vi "gyro -- async fitter.vi"(11 "server event pair":T9) -> ()   [LabVIEW 2020]
uses:
  lorentzian.ctl
  circle corners.ctl
  peak -- parameters -- complex fit.ctl
  wavepacket.ctl
  filter method control.ctl
  show-win- control.ctl
  server talk-to-back pair.ctl
  server talkback message type.ctl
  server talkto message type.ctl
  cwin.ctl
  plot refs -- filter related.ctl
  cursor window action.ctl
  publisher action.ctl
  cursor action.ctl
  2Dwindow.ctl
  filter - complex - four.vi
  linear interp iiii- complex - z-omega.vi
  peak -- PM find lorenzian - V3.vi
  tale of three indices.vi
  Q -- check range -- i -- real.vi
  filter -- window span logic.vi
  linear interp iiii- complex - z-omega - divide.vi
  linear interpolation iiii- complex.vi
  containing bix.vi
  <vilib>/Analysis/baseanly.llb/A x B.vi
  <vilib>/Analysis/baseanly.llb/Complex A x B.vi
  line -- complex.vi
  Q -- check range -- i -- integer.vi
  peak -- guess at omega -- dzdomega V2.vi
  command stack.vi
  tale of three indices -- check state.vi
  Q - not nan -- real.vi
  Q - not nan -- integer.vi
  peak -- z center from mult phase points.vi
  peak -- estimate for lorentzian.vi
  peak -- fake phase around center.vi
  peak -- get weights.vi
  peak -- four corner circle transformation logic.vi
  peak - fit phase around center - V2.vi
  array - generate range.vi
  circle center from three points.vi
  <vilib>/Utility/error.llb/Clear Errors.vi
  peak -- fit function -- minus arctan.vi
  <vilib>/Analysis/Matrix/Numeric/Conversions/Array To Matrix.vi
  <vilib>/Analysis/Matrix/Numeric/Conversions/Array To Matrix - RA2.vi
  <vilib>/Analysis/baseanly.llb/Inverse Matrix.vi
  <vilib>/Analysis/baseanly.llb/Real Inverse Matrix.vi
  <vilib>/gmath/NumericalOptimization/Nonlinear Curve Fit.vi
  <vilib>/gmath/NumericalOptimization/Nonlinear Curve Fit LM.vi
  KM_filter pipe - plot staff - more - V3.vi
panel:
  in  "Tab :  Fit controls":T1(tab)
  out "lorentzian":T2={"A (VHz)"=nan, "f (Hz)"=0.0, "G (Hz)"=0.0, "phi(rad)"=nan, "Q"=nan, "Norm  Ampl"=nan, "bg (V)"=nan+nani, "4corners"={"z (-pi/2)"=nan+nani, "z(inf)"=nan+nani, "z (pi/2)"=nan+nani, "z center"=nan+nani, "z(0)"=nan+nani, "radius"=nan}} {"bg (V)" format="%#9_9f"; "Q" format="%#9_9f"; "phi(rad)" format="%#9_9f"; "G (Hz)" format="%#9_9f"; "f (Hz)" format="%#9_9f"}
  in  "Plot: fragment - filter":cluster{dbl[], dbl[]}[](graph)=[{[], []}, {[], []}, {[], []}, {[], []}]
  out "Plot: phase around center":cluster{dbl[], dbl[]}[](graph)
  out "Plot: fragment":cluster{dbl[], dbl[]}[](graph)
  out "Plot: complex plane":cluster{dbl[], dbl[]}[](graph)=[{[], []}, {[nan, nan, nan, nan, nan, nan, nan, nan, nan, nan, nan, nan, nan, nan, nan, nan, nan, nan, nan, nan, nan, nan, nan, nan, nan, nan, nan, nan, nan, nan, nan, nan, nan, nan, nan, nan, nan, nan, nan, nan, nan, nan, nan, nan, nan, nan, nan, nan, nan, nan], [nan, nan, nan, nan, nan, nan, nan, nan, nan, nan, nan, nan, nan, nan, nan, nan, nan, nan, nan, nan, nan, nan, nan, nan, nan, nan, nan, nan, nan, nan, nan, nan, nan, nan, nan, nan, nan, nan, nan, nan, nan, nan, nan, nan, nan, nan, nan, nan, nan, nan]}, {[nan, nan, nan, nan, nan, nan, nan, nan, nan, nan, nan, nan, nan, nan, nan, nan, nan, nan, nan, nan], [nan, nan, nan, nan, nan, nan, nan, nan, nan, nan, nan, nan, nan, nan, nan, nan, nan, nan, nan, nan]}, {[nan, nan, nan, nan, nan, nan, nan, nan, nan, nan, nan, nan, nan, nan, nan, nan, nan, nan, nan, nan], [nan, nan, nan, nan, nan, nan, nan, nan, nan, nan, nan, nan, nan, nan, nan, nan, nan, nan, nan, nan]}, {[nan, nan, nan, nan, nan, nan, nan, nan, nan, nan, nan, nan, nan, nan, nan, nan, nan, nan, nan, nan], [nan, nan, nan, nan, nan, nan, nan, nan, nan, nan, nan, nan, nan, nan, nan, nan, nan, nan, nan, nan]}, {[nan, nan, nan, nan, nan, nan, nan, nan, nan, nan, nan, nan, nan, nan, nan, nan, nan, nan, nan, nan], [nan, nan, nan, nan, nan, nan, nan, nan, nan, nan, nan, nan, nan, nan, nan, nan, nan, nan, nan, nan]}, {[], []}]
  in  "scale gauge: Plot: complex plane":dbl(slide)=0.00275 min=0.0 max=0.3 step=1e-06 scale=1e-05..0.5 scale format="%#_3p"
  out "Plot: phase":cluster{"omega out":dbl[], dbl[]}(graph)
  out "Plot: win omega":T4(graph)
  out "Plot: dz/domega":cluster{"omega out":dbl[], dbl[]}(graph)
  in  "Plot: complex plane - filter":cluster{dbl[], dbl[]}[](graph)=[{[], []}, {[], []}, {[0.0, 0.0, 0.0, 0.0, 0.0, 0.0, 0.0, 0.0, 0.0, 0.0, 0.0, 0.0, 0.0, 0.0, 0.0, 0.0, 0.0, 0.0, 0.0, 0.0, 0.0, 0.0, 0.0, 0.0, 0.0, 0.0, 0.0, 0.0, 0.0, 0.0, 0.0, 0.0, 0.0, 0.0, 0.0, 0.0, 0.0, 0.0, 0.0, 0.0, 0.0, 0.0, 0.0, 0.0, 0.0, 0.0, 0.0, 0.0, 0.0, 0.0, 0.0, 0.0, 0.0, 0.0, 0.0, 0.0, 0.0, 0.0, 0.0, 0.0, 0.0, 0.0, 0.0, 0.0, 0.0, 0.0, 0.0, 0.0, 0.0, 0.0, 0.0, 0.0, 0.0, 0.0, 0.0, 0.0, 0.0, 0.0, 0.0, 0.0, 0.0, 0.0, 0.0, 0.0, 0.0, 0.0, 0.0, 0.0, 0.0, 0.0, 0.0, 0.0, 0.0, 0.0, 0.0, 0.0, 0.0, 0.0, 0.0, 0.0], [0.0, 0.0, 0.0, 0.0, 0.0, 0.0, 0.0, 0.0, 0.0, 0.0, 0.0, 0.0, 0.0, 0.0, 0.0, 0.0, 0.0, 0.0, 0.0, 0.0, 0.0, 0.0, 0.0, 0.0, 0.0, 0.0, 0.0, 0.0, 0.0, 0.0, 0.0, 0.0, 0.0, 0.0, 0.0, 0.0, 0.0, 0.0, 0.0, 0.0, 0.0, 0.0, 0.0, 0.0, 0.0, 0.0, 0.0, 0.0, 0.0, 0.0, 0.0, 0.0, 0.0, 0.0, 0.0, 0.0, 0.0, 0.0, 0.0, 0.0, 0.0, 0.0, 0.0, 0.0, 0.0, 0.0, 0.0, 0.0, 0.0, 0.0, 0.0, 0.0, 0.0, 0.0, 0.0, 0.0, 0.0, 0.0, 0.0, 0.0, 0.0, 0.0, 0.0, 0.0, 0.0, 0.0, 0.0, 0.0, 0.0, 0.0, 0.0, 0.0, 0.0, 0.0, 0.0, 0.0, 0.0, 0.0, 0.0, 0.0]}, {[0.0, 0.0, 0.0], [0.0, 0.0, 0.0]}, {[nan, nan, nan, nan, nan, nan, nan, nan, nan, nan, nan, nan, nan, nan, nan, nan, nan, nan, nan, nan], [nan, nan, nan, nan, nan, nan, nan, nan, nan, nan, nan, nan, nan, nan, nan, nan, nan, nan, nan, nan]}, {[0.0, 0.0, 0.0, 0.0, 0.0, 0.0, 0.0, 0.0, 0.0, 0.0, 0.0, 0.0, 0.0, 0.0, 0.0, 0.0, 0.0, 0.0, 0.0, 0.0], [0.0, 0.0, 0.0, 0.0, 0.0, 0.0, 0.0, 0.0, 0.0, 0.0, 0.0, 0.0, 0.0, 0.0, 0.0, 0.0, 0.0, 0.0, 0.0, 0.0]}]
  in  "parameters -- scan monitor control.ctlparameters: complex fit":T5={"main VI path"=path "", "scale factor"=3.0, "# of grid points"=200, "parameters: wavepacket"={"R"=0.5, "wave number"=22.0, "delta k"=7.0, "radii vector"=[], "radial section"=[], "wave vector"=22.0, "wavepacket is"=TRUE}, "span"=0.27789, "interference ?"=enum."cp z center", "filter method"=enum."three"} {"span" min=0.0 max=0.5 step=1e-05 scale=0.0001..0.5 scale format="%#_5f"; "parameters: wavepacket"."delta k" format="%#_3f"; "parameters: wavepacket"."wave number" format="%#_3f"; "parameters: wavepacket"."R" format="%#_3f"}
  in  "win":T8={"cen (Hz)"=45005.0594236074, "win (Hz)"=127.23590686512762, "left (Hz)"=44941.44147017484, "right (Hz)"=45068.67737703997}
  out "circle frequency (Hz)":dbl format="%#11_11f"
  out "circle gamma (Hz)":dbl format="%#11_11f"
  out "circle phase (rad)":dbl=nan format="%#11_11f"
  out "circle Q":dbl=nan format="%#11_11f"
  in  "use fast fit!":bool
  in  "plot staff!":enum16{"plot", "do not plot", "a"}(ring)
  in  "tab":enum32{"complex plane"}(tab)
  in  "Ignore win":T10={"cen (Hz)"=0.0, "win (Hz)"=0.0, "left (Hz)"=-8.969831627629043, "right (Hz)"=8.26461485679713}
  out "# of points":dbl=953.475933538175
  out "center (kHz)":dbl=3399.029286744401
  out "win width (kHz)":dbl=76.27809365793496
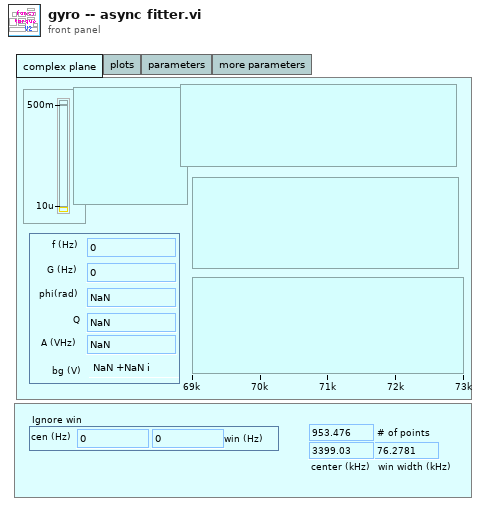
[diagram p1: front panel]
types:
  T1 = enum32{"complex plane", "plots", "parameters", "more parameters"}
  T2 = typedef "lorentzian.ctl" = cluster{"A (VHz)":dbl, "f (Hz)":dbl, "G (Hz)":dbl, "phi(rad)":dbl, "Q":dbl, "Norm  Ampl":dbl, "bg (V)":cdb, "4corners":T3}
  T3 = typedef "circle corners.ctl" = cluster{"z (-pi/2)":cdb, "z(inf)":cdb, "z (pi/2)":cdb, "z center":cdb, "z(0)":cdb, "radius":dbl}
  T4 = cluster{"omega out":dbl[], "win omega out":dbl[]}
  T5 = typedef "peak -- parameters -- complex fit.ctl" = cluster{"main VI path":path, "scale factor":dbl, "# of grid points":i32, "parameters: wavepacket":T6, "span":dbl, "interference ?":enum16{"cp z center", "pm zcenter", "fancy"}, "filter method":T7}
  T6 = typedef "wavepacket.ctl" = cluster{"R":dbl, "wave number":dbl, "delta k":dbl, "radii vector":dbl[], "radial section":cdb[], "wave vector":dbl, "wavepacket is":bool}
  T7 = typedef "filter method control.ctl" = enum16{"four", "five", "one", "two", "three", "zero", "minus one", "minus two"}
  T8 = typedef "show-win- control.ctl" = cluster{"cen (Hz)":dbl, "win (Hz)":dbl, "left (Hz)":dbl, "right (Hz)":dbl}
  T9 = typedef "server talk-to-back pair.ctl" = cluster{"talkback event":refnum<user-event>, "talkto event":refnum<user-event>}
  T10 = typedef "cwin.ctl" = cluster{"cen (Hz)":dbl, "win (Hz)":dbl, "left (Hz)":dbl, "right (Hz)":dbl}
  T11 = typedef "plot refs -- filter related.ctl" = cluster{"Plot: complex plane - filter":refnum<vi>, "Plot: dz/domega":refnum<vi>, "Plot: fragment filter":refnum<vi>, "Plot: win omega":refnum<vi>, "Plot: phase":refnum<vi>, "Plot: phase around center":refnum<vi>, "Plot: complex plane":refnum<vi>, "Plot: fragment":refnum<vi>}
  T12 = typedef "cursor window action.ctl" = enum16{"balance", "h. offset change", "cursor moves", "change center", "change window", "init", "check", "reset", "set y to middle", "idle", "-write all Y", "-write left.X", "-write center.X", "-write right.X", "-write all X", "-change center", "-change window", "-change skew", "-read cursor 2", "-read cursor 1", "-read cursor 0", "-read all cursors", "-reset", "-read plot scale", "-set y to middle", "-Q: center.Y is visible", "-Q: window is visible", "-parse center.Y", "-right left from center", "-left move", "-right move", "-set center.Y", "-empty", "-set cursors to default", "-check", "-write center.Y", "-copy cursor 1", "-copy cursor 0", "-copy cursor 2", "move right", "move left", "shrink", "broaden", "skew up", "skew down", "-write plot scale", "zoom X", "change cen&win", "zoom to all data", "color--red", "color--green", "color--yellow", "read", "zoom out", "zoom in", "slide right", "slide left", "set range aspect ratio to 1"}
  T13 = typedef "eventvkey.ctl" = enum16{"ASCII", "Enter", "Return", "Shift", "Ctrl", "Alt", "Cmd", "Opt", "Caps", "NumLock", "Clear", "Break", "Up", "Down", "Left", "Right", "Insert", "Delete", "Home", "End", "PageUp", "PageDown", "Escape", "Help", "Pause", "ScrollLock", "F1", "F2", "F3", "F4", "F5", "F6", "F7", "F8", "F9", "F10", "F11", "F12", "F13", "F14", "F15", "F16", "F17", "F18", "F19", "F20", "F21", "F22", "F23", "F24", "Play", "VolumeUp", "VolumeDown", "Mute", "Two Byte Char"}
  T14 = typedef "publisher action.ctl" = enum16{"set", "get", "init", "check"}
  T15 = typedef "server talkback message type.ctl" = cluster{"message":enum16{"new", "void"}}
  T16 = typedef "2Dwindow.ctl" = cluster{"window y":dbl, "center x":dbl, "center y":dbl, "window x":dbl}
  T17 = typedef "cursor action.ctl" = enum16{"range", "read", "write", "check", "zoom out", "smart zoom out", "zoom to aspect ratio 1", "zoom to win", "zoom out 20%", "zoom in 20%", "-empty", "smart zoom out&aspect", "move range left 20%", "move range right 20%", "move range up 20%", "move range down 20%", "zoom to X win", "zoom to Y win", "zoom out X", "zoom out Y", "zoom in X", "zoom in Y", "check plot scale"}
  T18 = typedef "cursor winow.ctl" = cluster{"left":dbl, "right ":dbl, "center":dbl, "window":dbl, "cursors":i32[], "relative":i32, "absolute":i32, "fixed vertical offset":dbl, "vertical offset":dbl, "skew":dbl, "default window frac":dbl, "kind":enum16{"symmetric", "skewed", "fancy"}, "skew.left":dbl, "skew.right":dbl, "Plot ref":refnum<vi>, "wing order":enum16{"forw", "back"}}
  T19 = enum16{"stop", "start", "update pars", "update request", "new", "launch", "exit", "get", "reset", "pause", "unpause"}
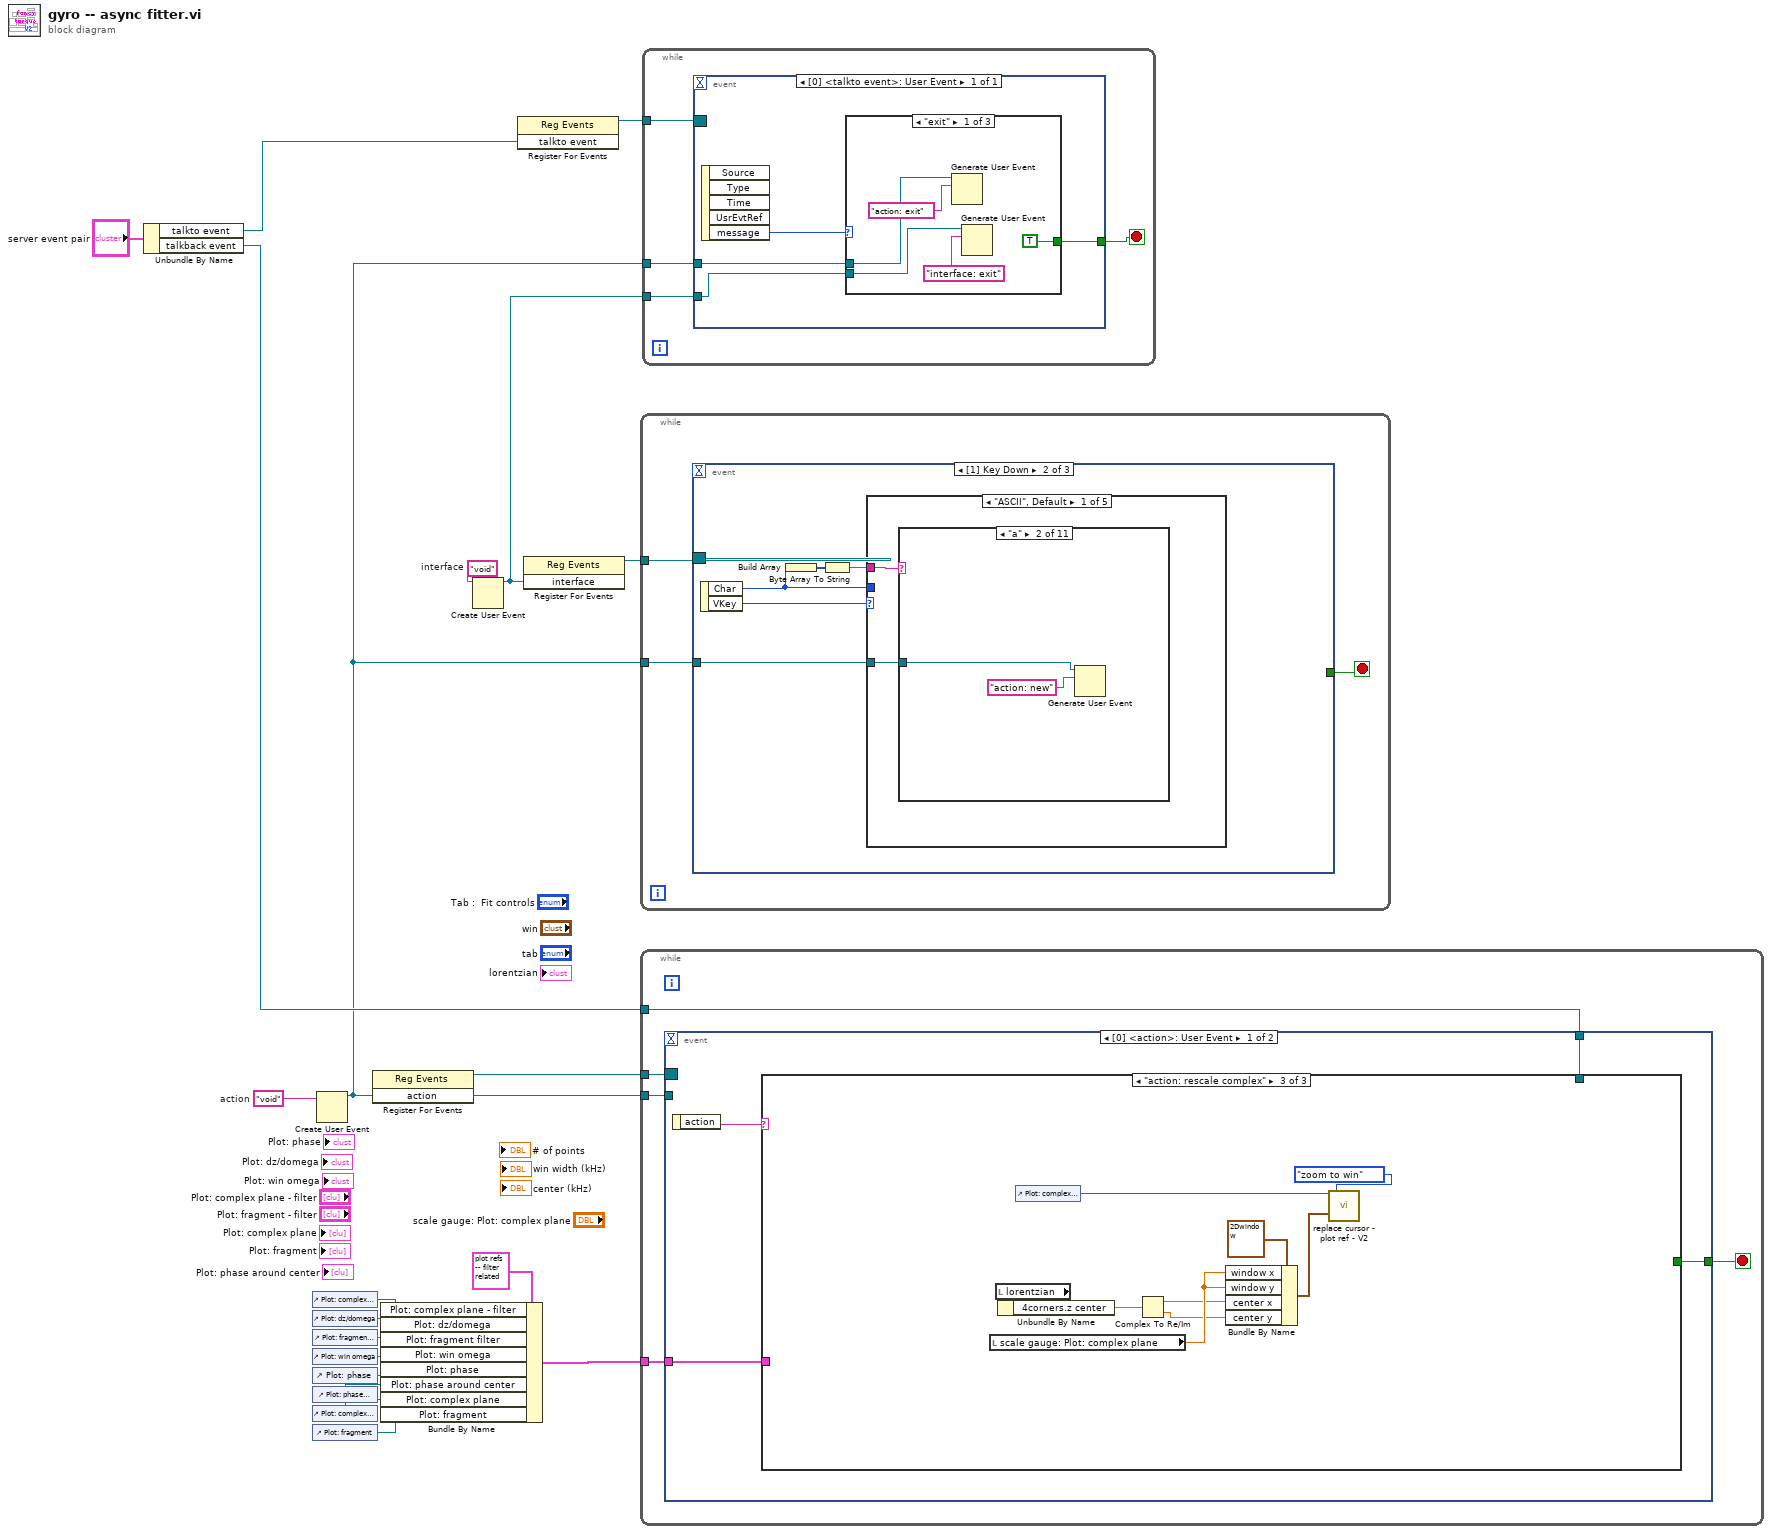
[diagram p0: block diagram]
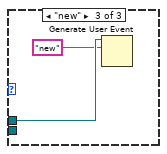
[diagram p3: hidden frame]
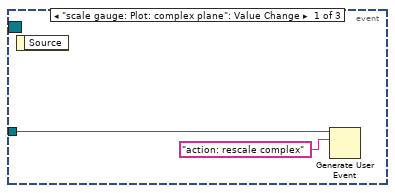
[diagram p4: hidden frame]
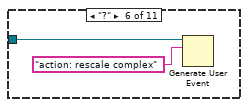
[diagram p9: hidden frame]
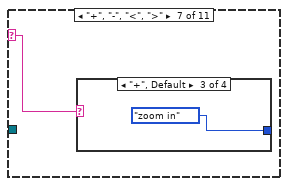
[diagram p10: hidden frame]
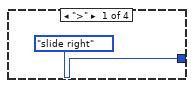
[diagram p11: hidden frame]
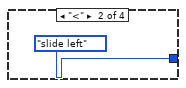
[diagram p12: hidden frame]
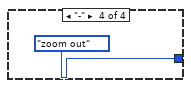
[diagram p13: hidden frame]
diagram:
  w17 = "void"  # interface
  w19 = "void"  # action
  n1 = Unbundle By Name("server event pair") -> ("talkto event"=w4:refnum<user-event>, "talkback event"=w3:refnum<user-event>)
  n2 = control-ref of="Plot: complex plane - filter"() -> (w15:refnum<vi>)
  n3 = control-ref of="Plot: dz/domega"() -> (w14:refnum<vi>)
  n4 = control-ref of="Plot: fragment - filter"() -> (w13:refnum<vi>)
  n5 = control-ref of="Plot: win omega"() -> (w12:refnum<vi>)
  n6 = control-ref of="Plot: phase"() -> (w11:refnum<vi>)
  n7 = control-ref of="Plot: phase around center"() -> (w9:refnum<vi>)
  n8 = control-ref of="Plot: complex plane"() -> (w8:refnum<vi>)
  n9 = control-ref of="Plot: fragment"() -> (w7:refnum<vi>)
  n10 = Create User Event(user event datatype=w19) -> (user event=w1:refnum<user-event>)  [unwired: 1 in, 1 out]
  n11 = register-events(w1) -> (reference out=w20:refnum<event-registration>)  [unwired: 2 in, 1 out]
  n12 = Bundle By Name(cluster=T11 {"Plot: complex plane - filter"=refnum, "Plot: dz/domega"=refnum, "Plot: fragment filter"=refnum, "Plot: win omega"=refnum, "Plot: phase"=refnum, "Plot: phase around center"=refnum, "Plot: complex plane"=refnum, "Plot: fragment"=refnum} ("plots: filter related"), "Plot: complex plane - filter"=w15, "Plot: dz/domega"=w14, "Plot: fragment filter"=w13, "Plot: win omega"=w12, "Plot: phase"=w11, "Plot: phase around center"=w9, "Plot: complex plane"=w8, "Plot: fragment"=w7) -> (w10:T11)
  n13 = Create User Event(user event datatype=w17) -> (user event=w2:refnum<user-event>)  [unwired: 1 in, 1 out]
  n14 = register-events(w4) -> (reference out=w6:refnum<event-registration>)  [unwired: 2 in, 1 out]
  n15 = register-events(w2) -> (reference out=w18:refnum<event-registration>)  [unwired: 2 in, 1 out]
  n16 = while {
    tunnel: w18 -> [w23]
    tunnel: w1 -> [w21]
    stop <- w22 stop-if-true
    n17 = event shown="[1] Key Down" {
      selector: w23 -> [_ _ _]
      dyn-events: _ -> [_ _ _]
      timeout: _ -> [_ _ _]
      tunnel: [_ _ w47] -> w22
      tunnel: w21 -> [w25 w26 _]
      event "scale gauge: Plot: complex plane": Value Change {
        n18 = event-data() -> ()  [unwired: 1 in, 1 out]
        n19 = Generate User Event(user event=w25, event data cluster="action: rescale complex" ("event data")) -> ()  [unwired: 2 in, 2 out]
      }
      event Key Down {
        n20 = event-data() -> ("Char"=w28:i16, "VKey"=w30:T13)  [unwired: 1 in]
        n21 = Build Array(w28) -> (w29:i16[])
        n22 = Byte Array To String(unsigned byte array=w29) -> (string=w27:string)
        n23 = case shown="\"ASCII\", Default" w30 {
          selector: w30 -> [_ _ _ _ w42]
          tunnel: w28 -> [_ _ _ _ _]
          tunnel: w27 -> [w32 _ _ _ _]
          tunnel: w26 -> [w31 _ _ _ _]
          frame "ASCII", Default {
            n24 = case shown="\"a\"" w32 {
              selector: w32 -> [_ _ _ _ _ _ w37 _ _ _ _]
              tunnel: w31 -> [_ w33 _ _ _ w35 _ _ _ _ _]
              frame "0", Default {
              }
              frame "a" {
                n25 = Generate User Event(user event=w33, event data cluster="action: new" ("event data")) -> ()  [unwired: 2 in, 2 out]
              }
              frame "s" {
              }
              frame "l" {
              }
              frame "p" {
              }
              frame "?" {
                n26 = Generate User Event(user event=w35, event data cluster="action: rescale complex" ("event data")) -> ()  [unwired: 2 in, 2 out]
              }
              frame "+", "-", "<", ">" {
                n27 = case shown="\"+\", Default" w37 {
                  tunnel: [cursor_window_action."slide right" ("cursor window action") cursor_window_action."slide left" ("cursor window action") cursor_window_action."zoom in" ("cursor window action") cursor_window_action."zoom out" ("cursor window action")] -> _
                  frame ">" {
                  }
                  frame "<" {
                  }
                  frame "+", Default {
                  }
                  frame "-" {
                  }
                }
              }
              frame "c" {
              }
              frame "t" {
              }
              frame "r" {
              }
              frame "d" {
              }
            }
          }
          frame "Escape" {
          }
          frame "PageUp" {
          }
          frame "PageDown" {
          }
          frame "Up".."Right" {
            n28 = case shown="\"Left\"" w42 {
              tunnel: [cursor_window_action."move right" ("cursor window action") cursor_window_action."move left" ("cursor window action") cursor_window_action."broaden" ("cursor window action") cursor_window_action."shrink" ("cursor window action")] -> _
              frame "Right", Default {
              }
              frame "Left" {
              }
              frame "Up" {
              }
              frame "Down" {
              }
            }
          }
        }
      }
      event User Event {
        n29 = event-data() -> ("interface"=w48:string)  [unwired: 1 in, 4 out]
        n30 = case shown="\"False\", Default" w48 {
          tunnel: [_ TRUE] -> w47
          frame "False", Default {
          }
          frame "interface: exit" {
          }
        }
      }
    }
  }
  n31 = while {
    tunnel: w20 -> [w54]
    tunnel: w1 -> [w53]
    tunnel: w10 -> [w52]
    tunnel: w3 -> [w51]
    stop <- w50 stop-if-true
    n32 = event shown="[0] <action>: User Event" {
      selector: w54 -> [_ _]
      dyn-events: _ -> [_ _]
      timeout: _ -> [_ _]
      tunnel: w53 -> [_ _]
      tunnel: w52 -> [w58 _]
      tunnel: w51 -> [w57 _]
      tunnel: [w55 _] -> w50
      event User Event {
        n33 = event-data() -> ("action"=w56:string)  [unwired: 1 in]
        n34 = case shown="\"action: rescale complex\"" w56 {
          tunnel: w58 -> [_ w61 _]
          tunnel: w57 -> [_ w60 _]
          tunnel: [TRUE _ _] -> w55
          frame "action: exit" {
          }
          frame "action: new", Default {
            n35 = flat-sequence {
              tunnel: w61 -> [w88]
              tunnel: w60 -> [w96]
              frame #0 {
                n36 = call "MFLI -- publish -- freq scan.vi"("publisher action"=publisher_action."get") -> ("Voltage out (V)"=w75:cdb[], "Freq out (Hz)"=w76:dbl[])  [unwired: 9 in]
                n37 = call "publish -- fitter window.vi"("publisher action"=publisher_action."get") -> ("win OUT"=w73:T18)  [unwired: 10 in]
                n38 = Unbundle By Name("Ignore win") -> ("cen (Hz)"=w64:dbl, "win (Hz)"=w67:dbl)
                n39 = call "acquire cursor window data.vi"("z in"=w75, "omega in"=w76, "cursor window"=w73) -> ("z out"=w71:cdb[], "omega  out"=w72:dbl[])  [unwired: 4 in, 3 out]
                n40 = Divide(x=w67, y=2.0) -> (x/y=w63:dbl)
                n41 = Subtract(x=w64, y=w63) -> (x-y=w62:dbl)
                n42 = Add(x=w64, y=w63) -> (x+y=w65:dbl)
                n43 = for {
                  tunnel: w72 -> [w93] mode=indexing
                  tunnel: w71 -> [w94] mode=indexing
                  tunnel: [w94] -> w69 mode=indexing if=w91
                  tunnel: [w93] -> w70 mode=indexing if=w91
                  tunnel: w65 -> [w90]
                  tunnel: w62 -> [w89]
                  n44 = In Range and Coerce(upper limit=w90, x=w93, lower limit=w89) -> (In Range?=w92:bool)  [unwired: 1 out]
                  n45 = Not(x=w92) -> (.not. x?=w91:bool)
                }
                n46 = call "KM_peak -- find -- pm - V1.vi"("omega in"=w70, "z in"=w69, "parameters: complex fit"="parameters -- scan monitor control.ctlparameters: complex fit", "plots: filter related"=w88, "plot staff ?"="plot staff!", "just guess?"="use fast fit!", "subtract linear BG"=FALSE) -> ("pm lorentzian"=w78:T2)  [unwired: 10 in, 2 out]
                n47 = Unbundle By Name(w78) -> ("f (Hz)"=→"circle frequency (Hz)":dbl, "G (Hz)"=→"circle gamma (Hz)":dbl, "phi(rad)"=→"circle phase (rad)":dbl, "Q"=→"circle Q":dbl)
                n48 = call "publish -- lorentzian.vi"("publisher action"=publisher_action."set", "lorentzian IN"=w78) -> ()  [unwired: 9 in, 1 out]
                n49 = local write "lorentzian"(w78) -> ()
              }
              frame #1 {
                n50 = Generate User Event(user event=w96, event data cluster=T15 {"message"=enum."new"} ("event data")) -> ()  [unwired: 2 in, 2 out]
              }
            }
          }
          frame "action: rescale complex" {
            n51 = local read "scale gauge: Plot: complex plane"() -> (w105:dbl)
            n52 = local read "lorentzian"() -> (w104:T2)
            n53 = Unbundle By Name(w104) -> ("4corners.z center"=w99:cdb)
            n54 = control-ref of="Plot: complex plane"() -> (w100:refnum<vi>)
            n55 = Complex To Re/Im(x + iy=w99) -> (x=w101:dbl, y=w102:dbl)
            n56 = Bundle By Name(cluster=T16 {"window y"=0.0021014740628288917, "center x"=44850.89441339177, "center y"=2.5658109925320947, "window x"=17480.201988350764} ("window IN"), "window x"=w105, "window y"=w105, "center x"=w101, "center y"=w102) -> (w103:T16)
            n57 = call "replace cursor - plot ref - V2.vi"("Plot ref in"=w100, "window IN"=w103, "cursor action"=cursor_action."zoom to win") -> ()  [unwired: 13 in, 4 out]
          }
        }
      }
      event Timeout {
        n58 = event-data() -> ()  [unwired: 1 in, 3 out]
      }
    }
  }
  n59 = while {
    tunnel: w6 -> [w109]
    tunnel: w1 -> [w107]
    tunnel: w2 -> [w106]
    stop <- w108 stop-if-true
    n60 = event shown="[0] <talkto event>: User Event" {
      selector: w109 -> [_]
      dyn-events: _ -> [_]
      timeout: _ -> [_]
      tunnel: [w112] -> w108
      tunnel: w107 -> [w111]
      tunnel: w106 -> [w110]
      event User Event {
        n61 = event-data() -> ("message"=w113:T19)  [unwired: 1 in, 4 out]
        n62 = case shown="\"exit\"" w113 {
          tunnel: [TRUE _ _] -> w112
          tunnel: w111 -> [w117 _ w120]
          tunnel: w110 -> [w114 _ _]
          frame "exit" {
            n63 = Generate User Event(user event=w117, event data cluster="action: exit" ("event data")) -> ()  [unwired: 2 in, 2 out]
            n64 = Generate User Event(user event=w114, event data cluster="interface: exit" ("event data")) -> ()  [unwired: 2 in, 2 out]
          }
          frame "start", Default {
          }
          frame "new" {
            n65 = Generate User Event(user event=w120, event data cluster="new" ("event data")) -> ()  [unwired: 2 in, 2 out]
          }
        }
      }
    }
  }
